vi "THD.vi"(8 "error in (no error)":errorcluster, 10 "distortion factor denominator":T1, 11 "harmonic spectra":T2(array[cluster])) -> (0 "error out":errorcluster, 2 "harmonic distortion factors [%]":dbl[][](array[numeric]), 3 "THD [%]":dbl[](array[numeric]), 4 "total values":dbl[](array[numeric]))   [LabVIEW 2013, in "NI_EP_Power Measurement.lvlib"]
doc: "Calculates the total harmonic distortion (THD), harmonic distortion factors, and total values from voltage harmonic spectra, current harmonic spectra, or harmonic spectra that contain both voltage and current."
uses:
  <vilib>/addons/Electrical Power/Power Measurement/NI_EP_Power Measurement.lvlib
  <vilib>/addons/Electrical Power/Power Measurement/subVIs/ep_Distortion Factor Denominator.ctl
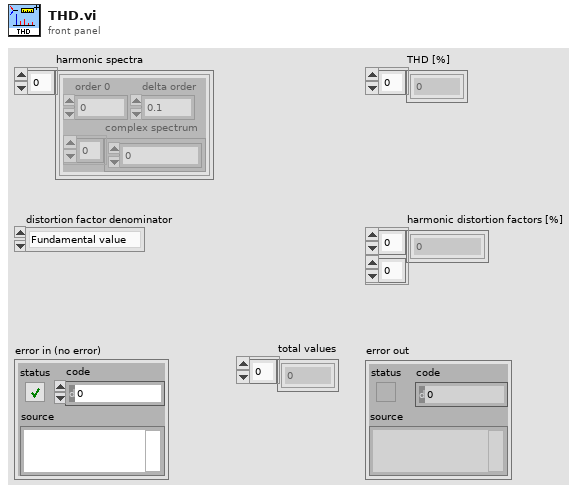
[diagram p1: front panel]
types:
  T1 = typedef "NI_EP_Power Measurement.lvlib/ep_Distortion Factor Denominator.ctl" = enum16{"Fundamental value", "Total value"}
  T2 = cluster{"order 0":dbl, "delta order":dbl, "complex spectrum":cdb[]}[]
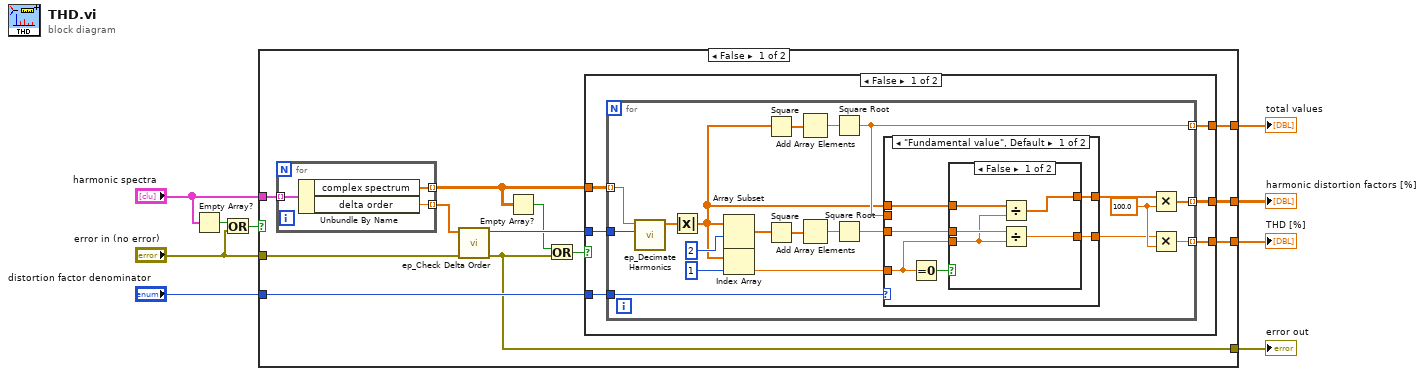
[diagram p0: block diagram]
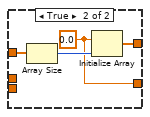
[diagram p2: hidden frame]
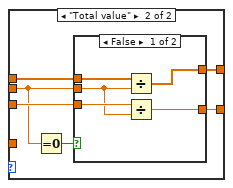
[diagram p3: hidden frame]
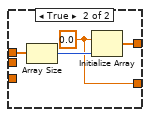
[diagram p4: hidden frame]
diagram:
  n1 = Empty Array?(array="harmonic spectra") -> (empty?=w4:bool)
  n2 = Or(x=w4, y="error in (no error)") -> (x .or. y?=w2:bool)
  n3 = case shown="False" w2 {
    tunnel: "harmonic spectra" -> [w16 _]
    tunnel: [w21 _] -> w9
    tunnel: "distortion factor denominator" -> [w20 _]
    tunnel: [w19 _] -> w8
    tunnel: [w14 w81] -> w7
    tunnel: [w17 _] -> w6
    tunnel: "error in (no error)" -> [w10 w81]
    frame False {
      n4 = for {
        tunnel: [w24] -> w12 mode=indexing
        tunnel: w16 -> [w23] mode=indexing
        tunnel: [w22] -> w15 mode=indexing
        n5 = Unbundle By Name(w23) -> ("complex spectrum"=w24:cdb[], "delta order"=w22:dbl)
      }
      n6 = call <vilib>:"ep_Check Delta Order.vi"("error in (no error)"=w10, "delta order"=w15) -> ("error out"=w14:errorcluster, "cycles per block"=w18:i32)  [unwired: 8 in]
      n7 = Empty Array?(array=w12) -> (empty?=w11:bool)
      n8 = Or(x=w11, y=w14) -> (x .or. y?=w13:bool)
      n9 = case shown="False" w13 {
        tunnel: w18 -> [w30 _]
        tunnel: [w29 _] -> w21
        tunnel: w20 -> [w28 _]
        tunnel: [w27 _] -> w19
        tunnel: w12 -> [w26 _]
        tunnel: [w25 _] -> w17
        frame False {
          n10 = for {
            tunnel: w30 -> [w42]
            tunnel: [w48] -> w29 mode=indexing
            tunnel: w28 -> [w35]
            tunnel: [w45] -> w27 mode=indexing
            tunnel: [w44] -> w25 mode=indexing
            tunnel: w26 -> [w33] mode=indexing
            w46 = 100.0
            n11 = call <vilib>:"ep_Decimate Harmonics.vi"("decimation factor"=w42, "array in"=w33) -> ("decimated array"=w41:cdb[])  [unwired: 9 in]
            n12 = Absolute Value(x=w41) -> (abs(x)=w34:dbl[])
            n13 = Array Subset(array=w34, index=2 ("y")) -> (w36:dbl[])  [unwired: 1 in]
            n14 = Index Array(array=w34, index=1) -> (element=w39:dbl)
            n15 = Square(x=w34) -> (x^2=w43:dbl[])
            n16 = Square(x=w36) -> (x^2=w37:dbl[])
            n17 = Add Array Elements(numeric array=w43) -> (sum=w50:dbl)
            n18 = Add Array Elements(numeric array=w37) -> (sum=w49:dbl)
            n19 = Square Root(x=w50) -> (sqrt(x)=w48:dbl)
            n20 = Square Root(x=w49) -> (sqrt(x)=w47:dbl)
            n21 = case shown="\"Fundamental value\", Default" w35 {
              tunnel: w34 -> [w56 w70]
              tunnel: w48 -> [_ w66]
              tunnel: w47 -> [w55 w67]
              tunnel: w39 -> [w52 _]
              tunnel: [w54 w69] -> w32
              tunnel: [w53 w68] -> w31
              frame "Fundamental value", Default {
                n22 = Equal To 0?(x=w52) -> (x = 0?=w51:bool)
                n23 = case shown="False" w51 {
                  tunnel: w56 -> [w61 w64]
                  tunnel: w55 -> [w60 _]
                  tunnel: [w59 w63] -> w54
                  tunnel: [w58 w62] -> w53
                  tunnel: w52 -> [w57 _]
                  frame False {
                    n24 = Divide(x=w61, y=w57) -> (x/y=w59:dbl[])
                    n25 = Divide(x=w60, y=w57) -> (x/y=w58:dbl)
                  }
                  frame True {
                    w62 = 0.0 ("vector")
                    n26 = Array Size(array=w64) -> (size(s)=w65:i32)
                    n27 = Initialize Array(w62, w65) -> (w63:dbl[])
                  }
                }
              }
              frame "Total value" {
                n28 = Equal To 0?(x=w66) -> (x = 0?=w71:bool)
                n29 = case shown="False" w71 {
                  tunnel: [w74 w79] -> w69
                  tunnel: [w76 w78] -> w68
                  tunnel: w70 -> [w75 w77]
                  tunnel: w67 -> [w73 _]
                  tunnel: w66 -> [w72 _]
                  frame False {
                    n30 = Divide(x=w75, y=w72) -> (x/y=w74:dbl[])
                    n31 = Divide(x=w73, y=w72) -> (x/y=w76:dbl)
                  }
                  frame True {
                    w78 = 0.0 ("vector")
                    n32 = Array Size(array=w77) -> (size(s)=w80:i32)
                    n33 = Initialize Array(w78, w80) -> (w79:dbl[])
                  }
                }
              }
            }
            n34 = Multiply(x=w32, y=w46) -> (x*y=w45:dbl[])
            n35 = Multiply(x=w31, y=w46) -> (x*y=w44:dbl)
          }
        }
        frame True {
        }
      }
    }
    frame True {
    }
  }
  "error out" <- w7
  "THD [%]" <- w6
  "total values" <- w9
  "harmonic distortion factors [%]" <- w8
